vi "Initialize.vi"(7 "Serial Configuration":T1={"Baud Rate"=9600, "Parity"=0, "Data Bits"=8, "Flow Control"=4} {"Flow Control" items=["None", "XON/XOFF", "RTS/CTS", "XON/XOFF & RTS/CTS", "DTR/DSR", "XON/XOFF & DTR/DSR"]; "Data Bits" items=["7"=7, "8"=8]; "Parity" items=["None", "Odd", "Even", "Mark", "Space"]; "Baud Rate" items=["300"=300, "600"=600, "1200"=1200, "2400"=2400, "4800"=4800, "9600"=9600, "19200"=19200]}, 8 "error in (no error)":errorcluster, 9 "Reset (True)":bool=TRUE, 10 "ID Query (True)":bool=TRUE, 11 "VISA resource name":refnum<visa-resource-name>) -> (0 "error out":errorcluster, 2 "idn string":string, 3 "VISA resource name out":refnum<visa-resource-name>)   [LabVIEW 2020, in "AWG.lvlib" / "Agilent 33XXX Series.lvlib"]
doc: "Establishes communication with the instrument and optionally performs an instrument identification query and/or an instrument reset. It also places the instrument in a default state needed for other instrument driver operations. Therefore, call this VI before calling other instrument driver VIs for this instrument. Generally, you need to call the <B>Initialize VI</B> only once at the beginning of an application."
uses:
  Agilent 33XXX Series.lvlib
panel:
  # "(c) 2005- 2013 National Instruments.  ALL RIGHTS RESERVED."
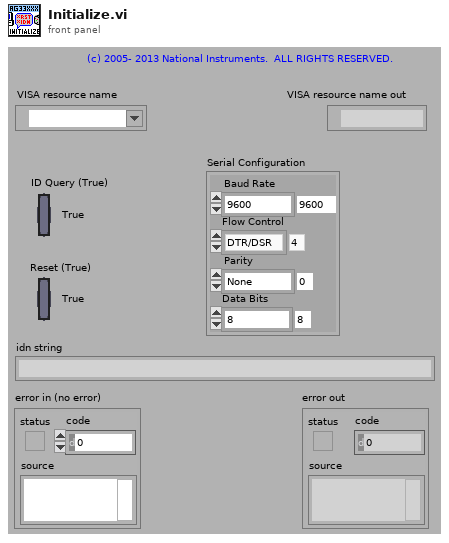
[diagram p1: front panel]
types:
  T1 = cluster{"Baud Rate":u32, "Parity":u16, "Data Bits":u16, "Flow Control":u16}
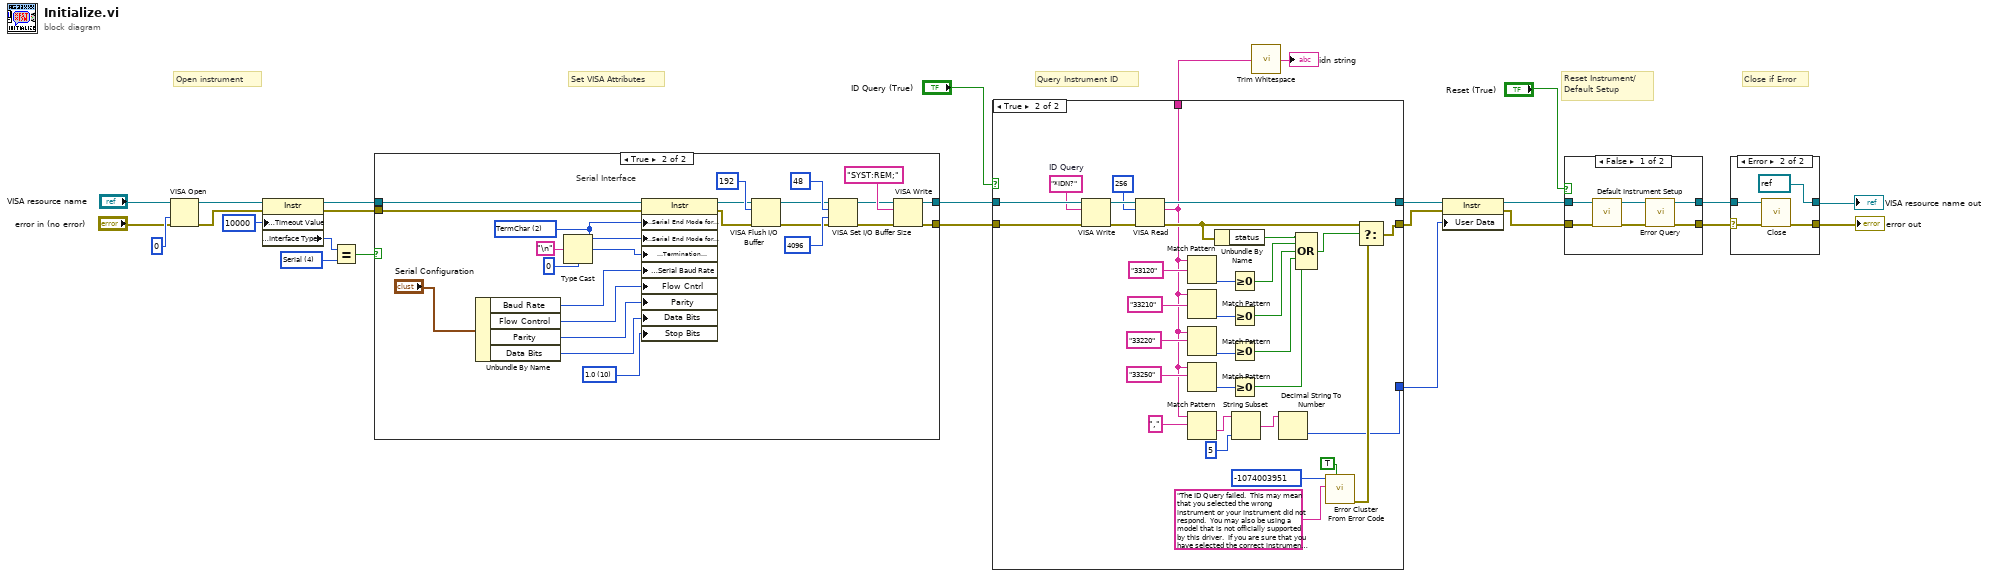
[diagram p0: block diagram]
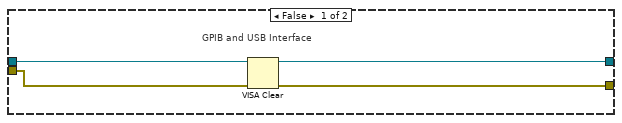
[diagram p2: hidden frame]
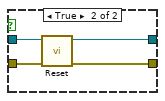
[diagram p4: hidden frame]
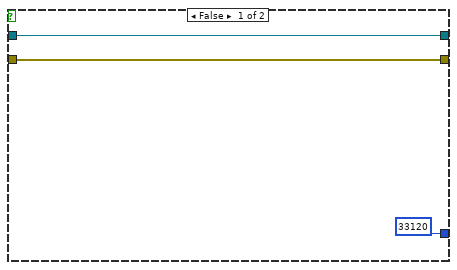
[diagram p5: hidden frame]
diagram:
  w19 = u16 4 items=["GPIB"=1, "VXI"=2, "GPIB-VXI"=3, "Serial"=4, "PXI"=5, "TCPIP"=6, "USB"=7] ("Interface Information:Interface Type")
  # "Set VISA Attributes"
  # "Close if Error"
  # "Query Instrument ID"
  # "Reset Instrument/\nDefault Setup"
  # "Open instrument"
  n1 = VISA Open(access mode=u32 0, error in (no error)="error in (no error)", VISA resource name="VISA resource name") -> (VISA resource name=w16:refnum<visa-resource-name>, error out=w15:errorcluster)  [unwired: 2 in]
  n2 = property class="Instr"(reference=w16, error in=w15, "General Settings:Timeout Value"=u32 10000) -> (reference out=w22:refnum<visa-resource-name>, error out=w21:errorcluster, "Interface Information:Interface Type"=w26:u16)
  n3 = Equal?(x=w26, y=w19) -> (x = y?=w20:bool)
  n4 = case shown="True" w20 {
    tunnel: [w28 w42] -> w24
    tunnel: [w27 w43] -> w23
    tunnel: w22 -> [w30 w53]
    tunnel: w21 -> [w29 w54]
    frame False {
      # "GPIB and USB Interface"
      n5 = VISA Clear(VISA resource name=w30, error in (no error)=w29) -> (VISA resource name out=w28:refnum<visa-resource-name>, error out=w27:errorcluster)
    }
    frame True {
      w32 = u16 10 items=["1.0"=10, "1.5"=15, "2.0"=20] ("Serial Settings:Stop Bits")
      w50 = u16 2 items=["None", "LastBit", "TermChar"] ("Serial Settings:Serial End Mode for Reads")
      # "Serial Interface"
      n6 = Unbundle By Name("Serial Configuration") -> ("Baud Rate"=w47:u32, "Flow Control"=w31:u16, "Parity"=w46:u16, "Data Bits"=w45:u16)
      n7 = Type Cast(type=u8 0, x="\n" ("Line Feed Constant")) -> (*(type *) &x=w49:u8)
      n8 = property class="Instr"(reference=w53, error in=w54, "Serial Settings:Serial End Mode for Reads"=w50, "Serial Settings:Serial End Mode for Writes"=w50, "Message Based Settings:Termination Character"=w49, "Serial Settings:Serial Baud Rate"=w47, "Flow Cntrl"=w31, "Parity"=w46, "Data Bits"=w45, "Stop Bits"=w32) -> (reference out=w40:refnum<visa-resource-name>, error out=w39:errorcluster)
      n9 = VISA Flush I/O Buffer(VISA resource name=w40, mask (16)=u16 192, error in (no error)=w39) -> (VISA resource name out=w35:refnum<visa-resource-name>, error out=w36:errorcluster)
      n10 = VISA Set I/O Buffer Size(VISA resource name=w35, mask (16)=u16 48, size (4096)=u32 4096 ("size (0)"), error in (no error)=w36) -> (VISA resource name out=w34:refnum<visa-resource-name>, error out=w33:errorcluster)
      n11 = VISA Write(VISA resource name=w34, write buffer="SYST:REM;", error in (no error)=w33) -> (VISA resource name out=w42:refnum<visa-resource-name>, error out=w43:errorcluster)  [unwired: 1 out]
    }
  }
  n12 = case shown="True" "ID Query (True)" {
    tunnel: [w56 w90] -> w13
    tunnel: [w57 w87] -> w14
    tunnel: w24 -> [w57 w88]
    tunnel: w23 -> [w56 w89]
    tunnel: [33120 w71] -> w10
    tunnel: [_ w58] -> w2
    frame False {
    }
    frame True {
      w82 = "*IDN?"  # ID Query
      n13 = VISA Write(VISA resource name=w88, write buffer=w82, error in (no error)=w89) -> (VISA resource name out=w86:refnum<visa-resource-name>, error out=w85:errorcluster)  [unwired: 1 out]
      n14 = VISA Read(VISA resource name=w86, byte count=u32 256, error in (no error)=w85) -> (VISA resource name out=w87:refnum<visa-resource-name>, read buffer=w58:string, error out=w70:errorcluster)  [unwired: 1 out]
      n15 = Match Pattern(string=w58, regular expression="33120") -> (offset past match=w84:i32)  [unwired: 1 in, 3 out]
      n16 = Match Pattern(string=w58, regular expression="33210") -> (offset past match=w64:i32)  [unwired: 1 in, 3 out]
      n17 = Match Pattern(string=w58, regular expression="33220") -> (offset past match=w63:i32)  [unwired: 1 in, 3 out]
      n18 = Match Pattern(string=w58, regular expression="33250") -> (offset past match=w67:i32)  [unwired: 1 in, 3 out]
      n19 = Match Pattern(string=w58, regular expression=",") -> (after substring=w73:string)  [unwired: 1 in, 3 out]
      n20 = Unbundle By Name(w70) -> ("status"=w69:bool)
      n21 = Greater Or Equal To 0?(x=w84) -> (x >= 0?=w68:bool)
      n22 = Greater Or Equal To 0?(x=w64) -> (x >= 0?=w66:bool)
      n23 = Greater Or Equal To 0?(x=w63) -> (x >= 0?=w62:bool)
      n24 = Greater Or Equal To 0?(x=w67) -> (x >= 0?=w61:bool)
      n25 = String Subset(string=w73, length (rest)=5 ("length (rest)")) -> (substring=w74:string)  [unwired: 1 in]
      n26 = Decimal String To Number(string=w74) -> (number=w71:i32)  [unwired: 2 in, 1 out]
      n27 = Compound Arithmetic op=OR(w69, w68, w66, w62, w61) -> (w65:bool)
      n28 = call <vilib>:"Error Cluster From Error Code.vi"("show call chain? (False)"=TRUE, "error message (\"\")"="The ID Query failed.  This may mean that you selected the wrong instrument or your instrument did not respond.  You may also be using a model that is not officially supported by this driver.  If you are sure that you have selected the correct instrument and it is responding, try disabling the ID Query." ("Source (VI Name)"), "error code (0)"=-1074003951 ("Code")) -> ("error out"=w81:errorcluster)  [unwired: 6 in]
      n29 = Select(t=w70, s=w65, f=w81) -> (s? t:f=w90:errorcluster)
    }
  }
  n30 = call <vilib>:"Trim Whitespace.vi"("string"=w2) -> ("trimmed string"=→"idn string":string)  [unwired: 1 in]
  n31 = property class="Instr"(reference=w14, error in=w13, "User Data"=w10) -> (reference out=w11:refnum<visa-resource-name>, error out=w12:errorcluster)
  n32 = case shown="False" "Reset (True)" {
    tunnel: w12 -> [w95 w97]
    tunnel: [w91 w100] -> w17
    tunnel: w11 -> [w96 w98]
    tunnel: [w92 w99] -> w18
    frame False {
      n33 = call "Default Instrument Setup.vi"("error in (no error)"=w95, "VISA resource name"=w96) -> ("error out"=w93:errorcluster, "VISA resource name out"=w94:refnum<visa-resource-name>)  [unwired: 8 in]
      n34 = call "Error Query.vi"("error in (no error)"=w93, "VISA resource name"=w94) -> ("error out"=w91:errorcluster, "VISA resource name out"=w92:refnum<visa-resource-name>)  [unwired: 6 in, 2 out]
    }
    frame True {
      n35 = call "Reset.vi"("error in (no error)"=w97, "VISA resource name"=w98) -> ("error out"=w100:errorcluster, "VISA resource name out"=w99:refnum<visa-resource-name>)  [unwired: 8 in]
    }
  }
  n36 = case shown="Error" w17 {
    selector: w17 -> [w101 w104]
    tunnel: w18 -> [w102 w105]
    tunnel: [w102 refnum<visa-resource-name> refnum ("VISA resource name out")] -> w7
    tunnel: [w101 w106] -> w6
    frame No Error {
    }
    frame Error {
      n37 = call "Close.vi"("error in (no error)"=w104, "VISA resource name"=w105) -> ("error out"=w106:errorcluster)  [unwired: 9 in]
    }
  }
  "VISA resource name out" <- w7
  "error out" <- w6
